vi "send.vi"(0 "内容标识":string, 1 "时标":string, 4 "发送":bool, 7 "内容说明（文件名）":string, 8 "帧内容":string, 11 "帧数":string, 15 "帧号":string) -> (6 "CRC32效验码输出":string, 10 "帧长":string, 13 "连接的字符串":string)   [LabVIEW 2016, in "数据传输系统-06.lvlib" / "自动更新.lvlib" / "TCP文件传输系统.lvlib" / "TCP发送文件.lvlib"]
panel:
  out "长度":i32
  in  "结束标志":string="END"
  in  "帧头":string="55AA"
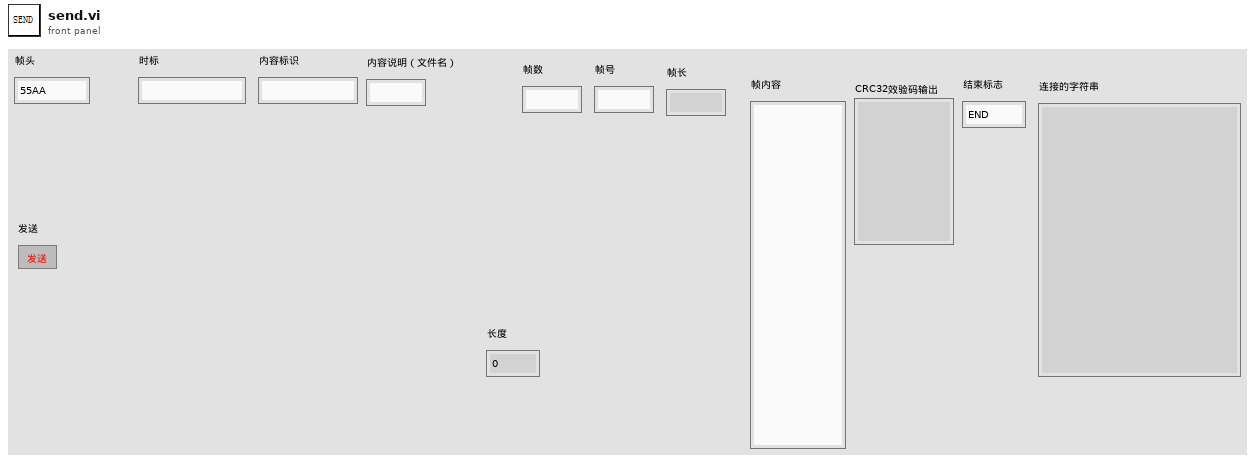
[diagram p1: front panel]
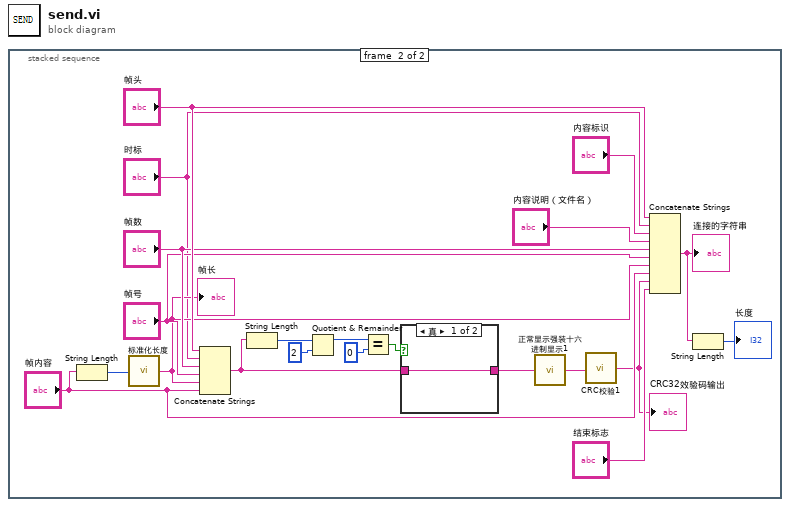
[diagram p0: block diagram]
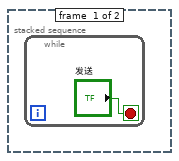
[diagram p2: hidden frame]
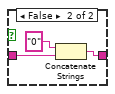
[diagram p3: hidden frame]
diagram:
  n1 = stacked-sequence {
    frame #0 {
      n2 = while {
        stop <- "发送" stop-if-true
      }
    }
    frame #1 {
      n3 = String Length(string="帧内容") -> (length=w19:i32)
      n4 = call "标准化长度.vi"("原长度"=w19) -> ("标准化长度"=w14:string)
      "帧长" <- w14
      n5 = Concatenate Strings("帧头", "时标", "帧数", "帧号", w14, "帧内容") -> (w9:string)
      n6 = String Length(string=w9) -> (length=w11:i32)
      n7 = Quotient & Remainder(x=w11, y=2) -> (x-y*floor(x/y)=w7:i32)  [unwired: 1 out]
      n8 = Equal?(x=w7, y=0) -> (x = y?=w5:bool)
      n9 = case shown="真" w5 {
        tunnel: [w23 w24] -> w4
        tunnel: w9 -> [w23 w25]
        frame True {
        }
        frame False {
          n10 = Concatenate Strings("0" ("字符串"), w25) -> (w24:string)
        }
      }
      n11 = call "正常显示强装十六进制显示1.vi"("正常格式显示字符串"=w4) -> ("十六进制格式显示"=w3:string)
      n12 = call "CRC校验1.vi"("要校验的字符串（十六进制显示）"=w3) -> ("CRC32效验码输出"=w2:string)
      "CRC32效验码输出" <- w2
      n13 = Concatenate Strings("帧头", "时标", "内容标识", "内容说明（文件名）", "帧数", "帧号", w14, "帧内容", w2, "结束标志") -> (w18:string)
      "连接的字符串" <- w18
      n14 = String Length(string=w18) -> (length=→"长度":i32)
    }
  }
